vi "Get Object Refs from Node.vi"(8 "error in (no error)":errorcluster, 10 "Refresh UI":T1, 11 "Data Value Reference in":T2) -> (0 "error out":errorcluster, 2 "Refresh UI out":T1, 3 "References":T3)   [LabVIEW 2017, in "J1939 editor node.lvclass"]
doc: "Gets the reference to the engine and a generic Module Editor Node reference from the node we have. This will be used for operations in the UI."
uses:
  J1939 editor node.lvclass
  <vilib>/NI/DCAF/Tag Editor Core/Table API/Table Manager/object ref.ctl
  <vilib>/NI/DCAF/Tag Editor Core/Configuration Editor/Classes/Engine Parent/Engine Parent Editor Node.lvclass
  <vilib>/NI/DCAF/Tag Editor Core/Configuration Editor/Classes/Module editor node/module editor node.lvclass
  <vilib>/NI/Configuration Framework/Node/NodeRef.ctl
  <vilib>/NI/Configuration Framework/Node/NISE_CEF_Node.lvclass
  <vilib>/NI/Configuration Framework/Node/RefreshUIEvent.ctl
  <vilib>/NI/DCAF/Tag Editor Core/Table API/Table Manager/Table Manager.lvclass
  <vilib>/NI/Module Execution Interface/Engine Configuration/engine configuration.lvclass
  module/configuration/J1939 configuration.lvclass
  <vilib>/NI/Configuration Framework/serializable configuration/NISE_CEF_serializable configuration.lvclass
  <vilib>/NI/Tag Bus Module Framework/channel/TBM channel.lvclass
  module/configuration/Line.ctl
  <vilib>/NI/Tag Bus/tag/Data Type.ctl
  <vilib>/NI/Tag Bus/tag/tag descriptor.lvclass
  <vilib>/NI/Tag Bus Module Framework/channel/channel classification.ctl
  C:/Program Files (x86)/National Instruments/LabVIEW 2017/vi.lib/NI/Configuration Framework/serializable configuration/NISE_CEF_serializable configuration.lvclass
  C:/Program Files (x86)/National Instruments/LabVIEW 2017/vi.lib/NI/DCAF/Tag Editor Core/Configuration Editor/Classes/Module editor node/module editor node.lvclass
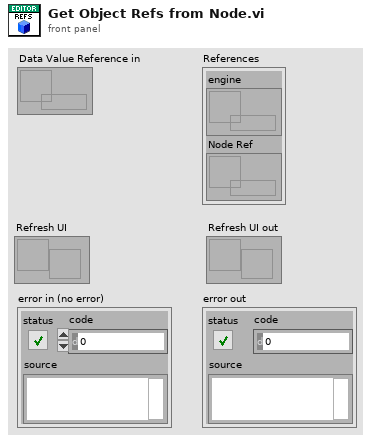
[diagram p1: front panel]
types:
  T1 = typedef "NISE_CEF_Node.lvclass/RefreshUIEvent.ctl" = refnum<user-event>
  T2 = typedef "NISE_CEF_Node.lvclass/NodeRef.ctl" = refnum<data-value>
  T3 = typedef "Table Manager.lvlib/Table Manager.lvclass/object ref.ctl" = cluster{"engine":refnum<data-value>, "Node Ref":refnum<data-value>}
  T4 = typedef "TBM channel.lvclass/channel classification.ctl" = enum16{"input data", "output data", "processing parameter", "processing result"}
  T5 = typedef "tag bus.lvlib/tag descriptor.lvclass/Data Type.ctl" = enum16{"Double", "Single", "I64", "I32", "I16", "I8", "U64", "U32", "U16", "U8", "Boolean", "String", "Array of Double", "Array of Single", "Array of I64", "Array of I32", "Array of I16", "Array of I8", "Array of U64", "Array of U32", "Array of U16", "Array of U8", "Array of Boolean", "Array of String"}
  T6 = typedef "J1939 configuration.lvclass/Line.ctl" = cluster{"channel":refnum<class "TBM channel.lvclass">, "XNET Signal":refnum<k21>}
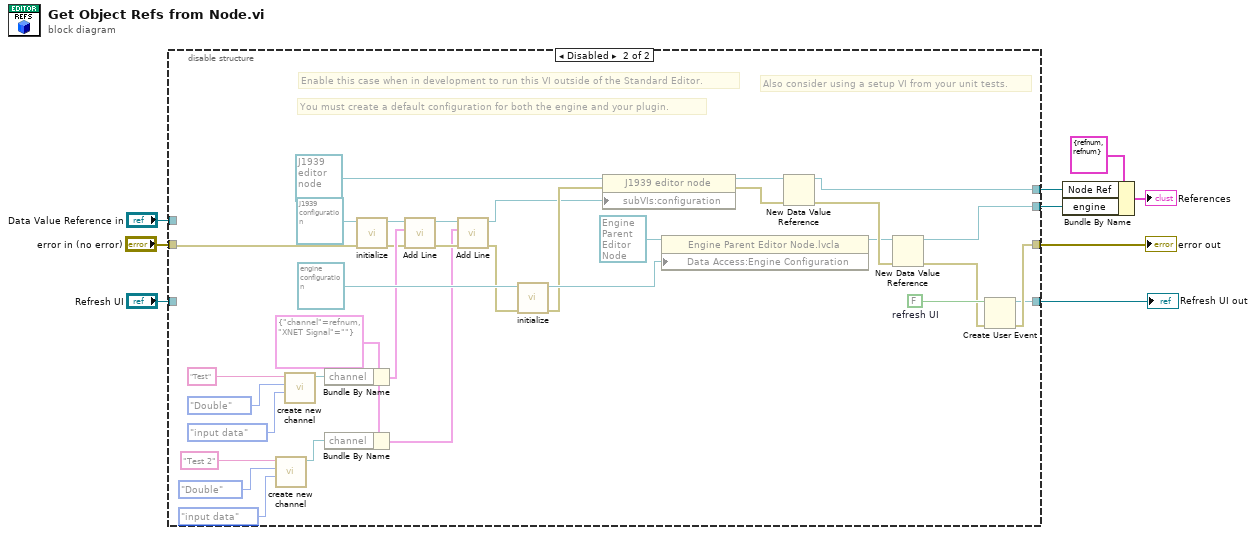
[diagram p0: block diagram]
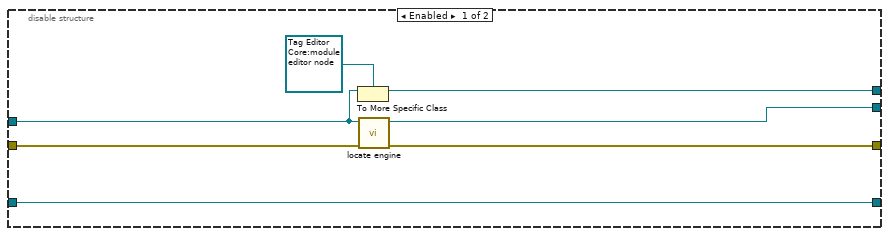
[diagram p2: hidden frame]
diagram:
  n1 = disable-structure shown="Disabled" {
    disable-tunnel: [w16 w40] -> w9
    disable-tunnel: "error in (no error)" -> [w15 w37]
    disable-tunnel: [w14 w42] -> w7
    disable-tunnel: "Data Value Reference in" -> [w13 _]
    disable-tunnel: [w11 w41] -> w4
    disable-tunnel: [w10 w39] -> w1
    disable-tunnel: "Refresh UI" -> [w10 _]
    frame Enabled {
      n2 = To More Specific Class(target class=refnum<data-value> refnum ("data value reference"), reference=w13) -> (specific class reference=w14:refnum<data-value>)  [unwired: 1 in, 1 out]
      n3 = call <vilib>:"locate engine.vi"("error in"=w15, "component"=w13) -> ("error out"=w16:errorcluster, "engine"=w11:refnum<data-value>)  [unwired: 8 in]
    }
    frame Disabled {
      w20 = T6 {"channel"=refnum, "XNET Signal"=""} ("Line")
      w48 = FALSE  # refresh UI
      # "Also consider using a setup VI from your unit tests."
      # "You must create a default configuration for both the engine and your plugin."
      # "Enable this case when in development to run this VI outside of the Standard Editor."
      n4 = call <vilib>:"create new channel.vi"("channel classification"=channel_classification."input data", "data type"=Data_Type."Double", "channel name"="Test 2") -> ("channel"=w23:refnum<class "TBM channel.lvclass">)  [unwired: 8 in]
      n5 = call <vilib>:"create new channel.vi"("channel classification"=channel_classification."input data", "data type"=Data_Type."Double", "channel name"="Test") -> ("channel"=w29:refnum<class "TBM channel.lvclass">)  [unwired: 8 in]
      n6 = Bundle By Name(cluster=w20, "channel"=w29) -> (w28:T6)
      n7 = Bundle By Name(cluster=w20, "channel"=w23) -> (w19:T6)
      n8 = call <vilib>:"initialize.vi"("error in"=w37, "configuration in"=refnum<class "J1939 configuration.lvclass"> refnum ("tag bus configurable plugin module configuration")) -> ("error out"=w27:errorcluster, "configuration out"=w33:refnum<class "J1939 configuration.lvclass">)  [unwired: 7 in, 1 out]
      n9 = call "Add Line.vi"("error in"=w27, "Line"=w28, "J1939 configuration in"=w33) -> ("error out"=w22:errorcluster, "J1939 configuration out"=w21:refnum<class "J1939 configuration.lvclass">)  [unwired: 6 in, 1 out]
      n10 = call "Add Line.vi"("error in"=w22, "Line"=w19, "J1939 configuration in"=w21) -> ("error out"=w18:errorcluster, "J1939 configuration out"=w17:refnum<class "J1939 configuration.lvclass">)  [unwired: 6 in, 1 out]
      n11 = call <vilib>:"initialize.vi"("error in"=w18, "configuration in"=refnum<class "engine configuration.lvclass"> refnum ("engine configuration")) -> ("error out"=w34:errorcluster, "configuration out"=w35:refnum<class "engine configuration.lvclass">)  [unwired: 7 in, 1 out]
      n12 = property class="J1939 editor node"(reference=refnum<class "J1939 editor node.lvclass"> refnum ("tag bus configurable plugin editor node"), error in=w34, "subVIs:configuration"=w17) -> (reference out=w44:refnum<class "J1939 editor node.lvclass">, error out=w50:errorcluster)
      n13 = property class="Engine Parent Editor Node.lvcla"(reference=refnum<class "Engine Parent Editor Node.lvclass"> refnum ("PL Framework Configuration Tool.lvlib:Engine Parent Editor Node.lvclass"), "Data Access:Engine Configuration"=w35) -> (reference out=w45:refnum<class "Engine Parent Editor Node.lvclass">)  [unwired: 1 in, 1 out]
      n14 = New Data Value Reference(data value=w44, error in=w50) -> (data value reference=w42:refnum<data-value>, error out=w49:errorcluster)
      n15 = New Data Value Reference(data value=w45, error in=w49) -> (data value reference=w41:refnum<data-value>, error out=w47:errorcluster)
      n16 = Create User Event(user event datatype=w48, error in=w47) -> (user event=w39:refnum<user-event>, error out=w40:errorcluster)
    }
  }
  "error out" <- w9
  "Refresh UI out" <- w1
  n17 = Bundle By Name(cluster=T3 {"engine"=refnum, "Node Ref"=refnum} ("references"), "Node Ref"=w7, "engine"=w4) -> (→"References":T3)
